vi "Reset Aisle of Records.vi"(0 "GUI Aisle In":T1[](array[typedef]) {"Night Cycle Count" format="%04d"; "Day Cycle Count" format="%05d"}) -> (4 "Aisle Array Out":T1[](array[typedef]) {"Night Cycle Count" format="%04d"; "Day Cycle Count" format="%05d"})   [LabVIEW 2011]
uses:
  Dryer.ctl
  Dryer Details.ctl
  Update Wilt GUI Control.ctl
panel:
  in  "Day Shift?":bool
  # "D"
  # "N"
  # "D"
  # "N"
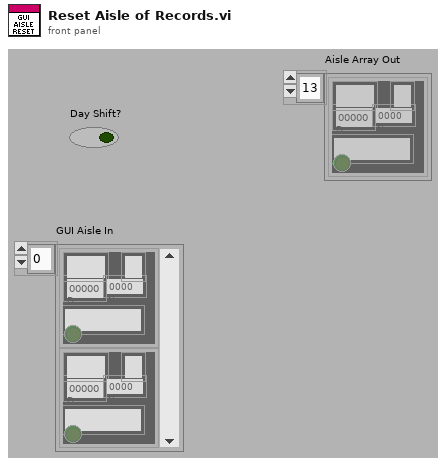
[diagram p1: front panel]
types:
  T1 = typedef "Dryer.ctl" = cluster{"Serial Number":string, "Day Cycle Count":i32, "Station Label":string, "Dryer Details":T2, "Sample Record(t, CC, Tc, ASCII, Status, L1,L2,Trmb,V{,V2,SW} ) ":string[], "Hist Record(Cycle Count, t-comp,L1max, L2max, Tmax) ":string[][], "Status Color":u32, "Boolean":bool, "Com Port":u8, "Bad Com Count":i32, "Current Run Start Time":dbl, "Night Cycle Count":i32, "Station Index":i32, "Cycle Index":string, "Audit Alert":bool}
  T2 = typedef "Dryer Details.ctl" = cluster{"Station":string, "Cycle Count Day":string, "Status":string, "Debug ASCII":string, "Notes":string, "Serial Number":string, "Total Time On":string, "TR Number":string, "Cycle Count Night":string, "Time On Day":string, "Time On Night":string}
  T3 = typedef "Update Wilt GUI Control.ctl" = enum16{"Init Station Number", "Update Detail Data", "Update Status", "Init Com Port Num", "Update Sample Info", "Reset All Cycles"}
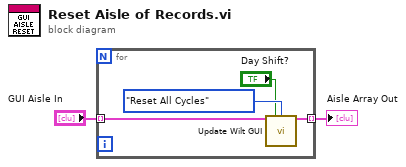
[diagram p0: block diagram]
diagram:
  n1 = for {
    tunnel: "GUI Aisle In" -> [w6] mode=indexing
    tunnel: [w5] -> w2 mode=indexing
    n2 = call "Update Wilt GUI.vi"("Dryer In"=w6, "Day Shift?"="Day Shift?", "Enum"=Update_Wilt_GUI_Control."Reset All Cycles") -> ("Dryer Out"=w5:T1)  [unwired: 10 in, 2 out]
  }
  "Aisle Array Out" <- w2
